vi "Read.vi"(8 "error in (no error)":errorcluster, 10 "byte count":u32, 11 "Serial Logging Decorator in":refnum<class "Serial Logging Decorator.lvclass">) -> (0 "error out":errorcluster, 2 "read buffer":string, 3 "Serial Logging Decorator out":refnum<class "Serial Logging Decorator.lvclass">)   [LabVIEW 2020, in "Serial Logging Decorator.lvclass"]
uses:
  Serial Logging Decorator.lvclass
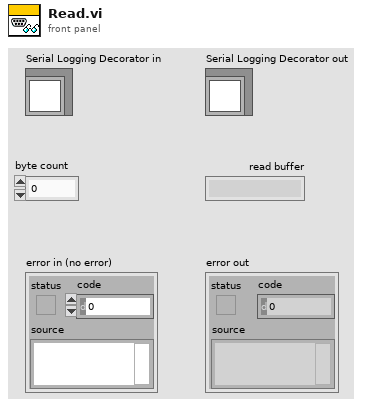
[diagram p1: front panel]
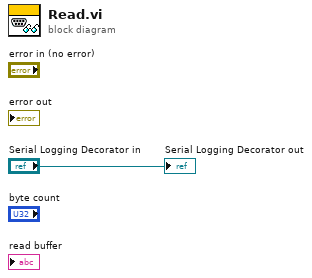
[diagram p0: block diagram]
diagram:
  "Serial Logging Decorator out" <- "Serial Logging Decorator in"
